vi "MB Auswahl Beschreiben.vi"(7 "Auswahl Referenz":refnum<vi>, 8 "NUR STRINGS?":bool, 10 "Komponente":i32) -> ()   [LabVIEW 2020, in "Analysator Definition.lvlib"]
doc: "0...........FTIR\n1...........PMA\n2...........FID CH4\n3...........FID THC\n4...........FID NMHC"
uses:
  Analysator Definition.lvlib
  Visualisierungs Elemente/Auswahlfeld.ctl
  FGV Analysator Definition Aktionen.ctl
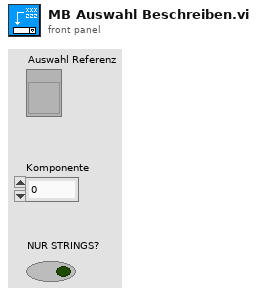
[diagram p1: front panel]
types:
  T1 = typedef "Analysator Definition.lvlib/FGV Analysator Definition Aktionen.ctl" = enum16{"lesen", "MB setzen", "MB KAL setzen", "laden"}
  T2 = typedef "Analysator Definition.lvlib/Betriebsdaten Komponente.ctl" = cluster{"Namen":string[], "MB Namen":string[], "Einheit":string, "MB Aktuell":u16, "MB Endwert":u16, "CalGase":u16[], "MB für KAL":u16[], "CG für KAL":u16[]}
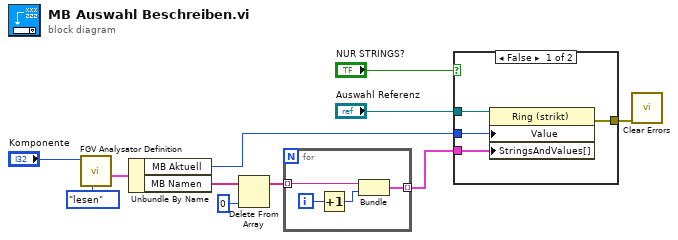
[diagram p0: block diagram]
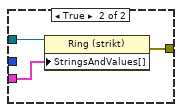
[diagram p2: hidden frame]
diagram:
  n1 = call "FGV Analysator Definition.vi"("Aktionen"=FGV_Analysator_Definition_Aktionen."lesen", "Komponente"="Komponente") -> ("Betriebsdaten Komponente"=w10:T2)  [unwired: 5 in, 4 out]
  n2 = Unbundle By Name(w10) -> ("MB Aktuell"=w3:u16, "MB Namen"=w9:string[])
  n3 = Delete From Array(array=w9, index=0 ("Index")) -> (array with subset deleted=w5:string[])  [unwired: 1 in, 1 out]
  n4 = for {
    tunnel: w5 -> [w14] mode=indexing
    tunnel: [w12] -> w4 mode=indexing
    i -> [w15]
    n5 = Increment(x=w15) -> (x+1=w13:i32)
    n6 = Bundle("MB"=w14, w13) -> (w12:cluster{"MB":string, i32})  [unwired: 1 in]
  }
  n7 = case shown="False" "NUR STRINGS?" {
    tunnel: "Auswahl Referenz" -> [w19 w20]
    tunnel: w4 -> [w18 w22]
    tunnel: w3 -> [w17 _]
    tunnel: [w16 w21] -> w2
    frame False {
      n8 = property class="Ring (strikt)"(reference=w19, "Value"=w17, "StringsAndValues[]"=w18) -> (error out=w16:errorcluster)  [unwired: 1 in, 1 out]
    }
    frame True {
      n9 = property class="Ring (strikt)"(reference=w20, "StringsAndValues[]"=w22) -> (error out=w21:errorcluster)  [unwired: 1 in, 1 out]
    }
  }
  n10 = call <vilib>:"Clear Errors.vi"("error in (no error)"=w2) -> ()  [unwired: 5 in, 2 out]
